vi "GetPhysChannel.vi"(8 "error in (no error)":errorcluster, 11 "Subsystem in":refnum<class "DAQmx(AI).lvclass">) -> (0 "error out":errorcluster, 2 "PhysChan":tag="SMO-Sim/ai0", 3 "Subsystem out":refnum<class "DAQmx(AI).lvclass">, 5 "period (ms)":i64=50)   [LabVIEW 2013, in "DAQmx(AI).lvclass"]
uses:
  DAQmx(AI).lvclass
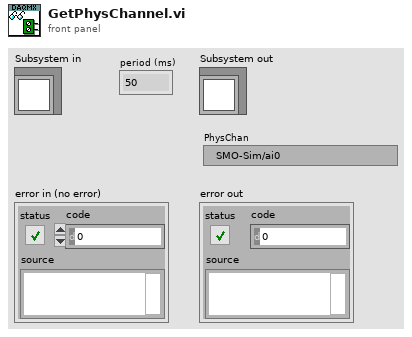
[diagram p1: front panel]
types:
  T1 = typedef "DAQmx(AI).lvclass/Configuration--Cluster.ctl" = cluster{"PhysChan":tag, "Period (ms)":i64, "input terminal cfg":i32, "minimum value":dbl, "maximum value":dbl, "units":T2, "task name":string}
  T2 = typedef "DAQmx(AI).lvclass/Units -- Enum.ctl" = enum16{"Volts", "Amps", "Deg F", "Deg C", "Deg R", "Kelvins", "Strain", "Ohms", "Hz", "Seconds", "Meters", "Inches", "Degrees", "Radians", "Ticks", "g", "m/s^2", "m/s", "in/s", "Pascals", "Newtons", "Pounds", "kgf", "psi", "bar", "Nm", "oz-in", "lb-in", "lb-ft", "Volts/Volt", "mVolts/Volt", "From TEDS"}
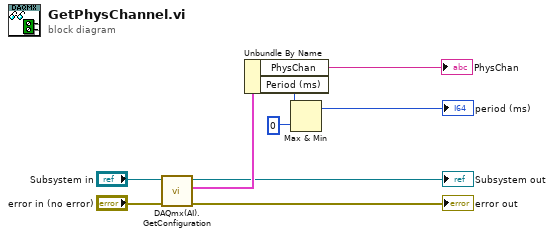
[diagram p0: block diagram]
diagram:
  n1 = call "DAQmx(AI).GetConfiguration.vi"("error in (no error)"="error in (no error)", "Subsystem"="Subsystem in") -> ("error out"=→"error out":errorcluster, "Configuration"=w9:T1, "Subsystem out"=→"Subsystem out":refnum<class "DAQmx(AI).lvclass">)  [unwired: 7 in]
  n2 = Unbundle By Name(w9) -> ("PhysChan"=→"PhysChan":tag, "Period (ms)"=w6:i64)
  n3 = Max & Min(x=w6, y=i64 0) -> (max(x,y)=→"period (ms)":i64)  [unwired: 1 out]
